vi "Config Delete Key.vi"(7 "Section Name":string, 8 "error in":errorcluster, 10 "Key Name":string, 11 "Config Cluster in":T1) -> (0 "error out":errorcluster, 2 "Found?":bool, 3 "Config Cluster out":T1)   [LabVIEW 2017]
uses:
  Config Cluster.ctl
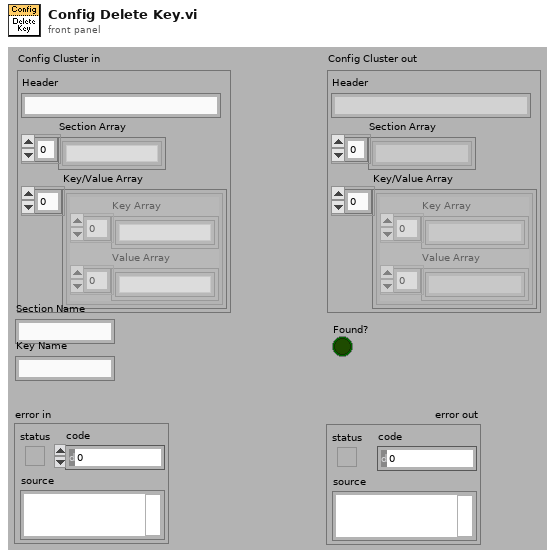
[diagram p1: front panel]
types:
  T1 = typedef "Config Cluster.ctl" = cluster{"Header":string, "Section Array":string[], "Key/Value Array":cluster{"Key Array":string[], "Value Array":string[]}[]}
  T2 = cluster{"Key Array":string[], "Value Array":string[]}[]
  T3 = cluster{"Key Array":string[], "Value Array":string[]}
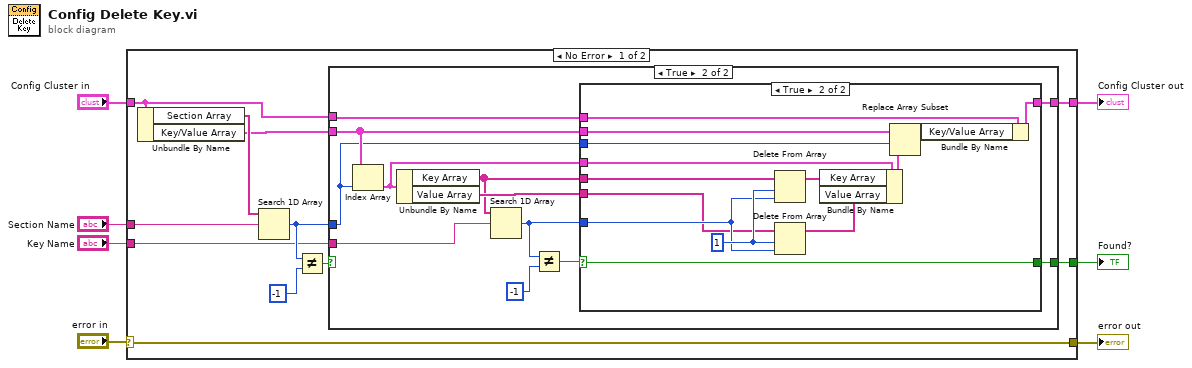
[diagram p0: block diagram]
diagram:
  n1 = case shown="No Error" "error in" {
    selector: "error in" -> [w9 w50]
    tunnel: [w9 w50] -> w6
    tunnel: "Config Cluster in" -> [w15 w49]
    tunnel: [w11 w49] -> w4
    tunnel: "Section Name" -> [w18 _]
    tunnel: "Key Name" -> [w10 _]
    tunnel: [w8 _] -> w1
    frame No Error {
      n2 = Unbundle By Name(w15) -> ("Section Array"=w13:string[], "Key/Value Array"=w12:T2)
      n3 = Search 1D Array(1D array=w13, element=w18) -> (index of element=w14:i32)  [unwired: 1 in]
      n4 = Not Equal?(x=w14, y=-1) -> (x != y?=w16:bool)
      n5 = case shown="True" w16 {
        selector: w16 -> [w19 _]
        tunnel: w15 -> [w20 w26]
        tunnel: w14 -> [_ w22]
        tunnel: w12 -> [_ w23]
        tunnel: [w20 w25] -> w11
        tunnel: w10 -> [_ w31]
        tunnel: [w19 w21] -> w8
        frame False {
          # "Section not found, nothing is deleted, Found? = F."
        }
        frame True {
          n6 = Index Array(array=w23, index=w22) -> (element=w24:T3)
          n7 = Unbundle By Name(w24) -> ("Key Array"=w27:string[], "Value Array"=w28:string[])
          n8 = Search 1D Array(1D array=w27, element=w31) -> (index of element=w29:i32)  [unwired: 1 in]
          n9 = Not Equal?(x=w29, y=-1) -> (x != y?=w30:bool)
          n10 = case shown="True" w30 {
            selector: w30 -> [w33 w35]
            tunnel: w29 -> [_ w47]
            tunnel: w28 -> [_ w45]
            tunnel: w27 -> [_ w46]
            tunnel: w26 -> [w34 w44]
            tunnel: [w34 w43] -> w25
            tunnel: w24 -> [_ w42]
            tunnel: w23 -> [_ w39]
            tunnel: w22 -> [_ w38]
            tunnel: [w33 w35] -> w21
            frame False {
              # "Key not found, nothing is deleted, Found? = F."
            }
            frame True {
              w48 = 1
              n11 = Delete From Array(array=w46, length=w48, index=w47) -> (array with subset deleted=w41:string[])  [unwired: 1 out]
              n12 = Delete From Array(array=w45, length=w48, index=w47) -> (array with subset deleted=w40:string[])  [unwired: 1 out]
              n13 = Bundle By Name(cluster=w42, "Key Array"=w41, "Value Array"=w40) -> (w37:T3)
              n14 = Replace Array Subset(array=w39, new element=w37, index=w38) -> (w36:T2)
              n15 = Bundle By Name(cluster=w44, "Key/Value Array"=w36) -> (w43:T1)
            }
          }
        }
      }
    }
    frame Error {
    }
  }
  "error out" <- w6
  "Config Cluster out" <- w4
  "Found?" <- w1
